vi "GetTandPNow.vi"(9 "Pressure channel":string, 10 "Temperature channel":string, 11 "History (s)":dbl) -> (1 "Press (mBar)":dbl, 2 "Temp (C)":dbl)   [LabVIEW 2016]
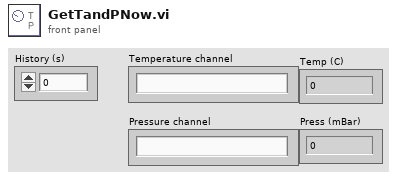
[diagram p1: front panel]
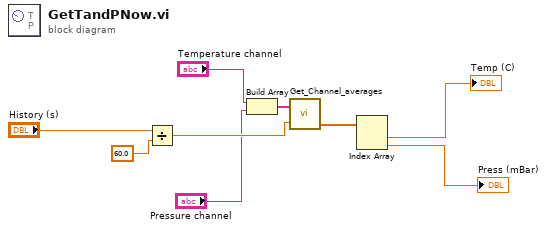
[diagram p0: block diagram]
diagram:
  n1 = Divide(x="History (s)", y=60.0 ("Averaging time (mins)")) -> (x/y=w9:dbl)
  n2 = Build Array("Temperature channel", "Pressure channel") -> (w1:string[])
  n3 = call "Get_Channel_averages.vi"("Desired Ch Names"=w1, "Averaging time (mins)"=w9) -> ("number"=w2:dbl[])  [unwired: 1 in, 2 out]
  n4 = Index Array(array=w2) -> (element #1=→"Temp (C)":dbl, element #2=→"Press (mBar)":dbl)  [unwired: 2 in]
